vi "Insert_Array_Subset.vi"(1 "String Array In":string[](array[string]), 2 "Array Subset":string[](array[string]), 3 "Subset Name":string) -> (0 "String Array Out":string[](array[string]))   [LabVIEW 2010]
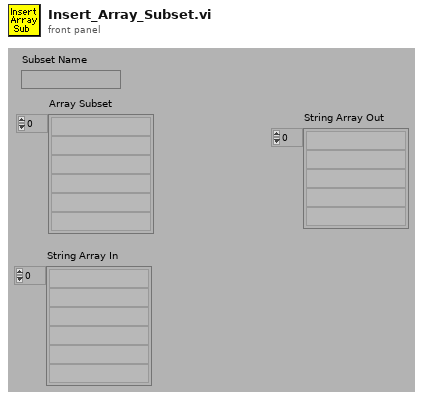
[diagram p1: front panel]
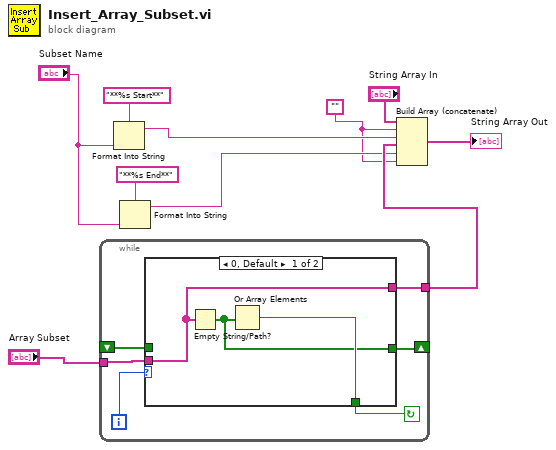
[diagram p0: block diagram]
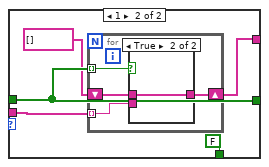
[diagram p2: hidden frame]
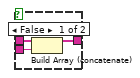
[diagram p3: hidden frame]
diagram:
  w1 = ""
  n1 = while {
    shift-left: _ -> [w11]
    shift-right: [w12] -> _
    tunnel: [w13] -> w5
    tunnel: "Array Subset" -> [w15]
    i -> [w16]
    stop <- w14 continue-if-true
    n2 = case shown="0, Default" w16 {
      tunnel: w15 -> [w18 w21]
      tunnel: [w19 FALSE] -> w14
      tunnel: [w18 w24] -> w13
      tunnel: [w17 w23] -> w12
      tunnel: w11 -> [_ w23]
      frame 0, Default {
        n3 = Empty String/Path?(string/path=w18) -> (empty?=w17:bool[])
        n4 = Or Array Elements(Boolean array=w17) -> (logical OR=w19:bool)
      }
      frame 1 {
        n5 = for {
          shift-right: [w27] -> w24
          shift-left: string[] [] -> [w26]
          tunnel: w23 -> [w28] mode=indexing
          tunnel: w21 -> [w25] mode=indexing
          n6 = case shown="True" w28 {
            tunnel: [w30 w32] -> w27
            tunnel: w26 -> [w31 w32]
            tunnel: w25 -> [w29 _]
            frame False {
              n7 = Build Array (concatenate)(w31, w29) -> (w30:string[])
            }
            frame True {
            }
          }
        }
      }
    }
  }
  n8 = Format Into String(format string="**%s Start**" ("Format String"), "Subset Name") -> (resulting string=w2:string)  [unwired: 2 in, 1 out]
  n9 = Format Into String(format string="**%s End**" ("Format String"), "Subset Name") -> (resulting string=w3:string)  [unwired: 2 in, 1 out]
  n10 = Build Array (concatenate)("String Array In", w1, w2, w5, w3, w1) -> (→"String Array Out":string[])
